vi "process waveplate positions.vi"(8 "error in (no error)":errorcluster, 11 "Channel in":refnum<class "SPARC4_Channel.lvclass">) -> (0 "error out":errorcluster, 3 "Channel out":refnum<class "SPARC4_Channel.lvclass">)   [LabVIEW 2018, in "SPARC4_Channel.lvclass"]
uses:
  SPARC4_Channel.lvclass
  SPARC4_Channel.lvclass/SPARC4_Channel.ctl
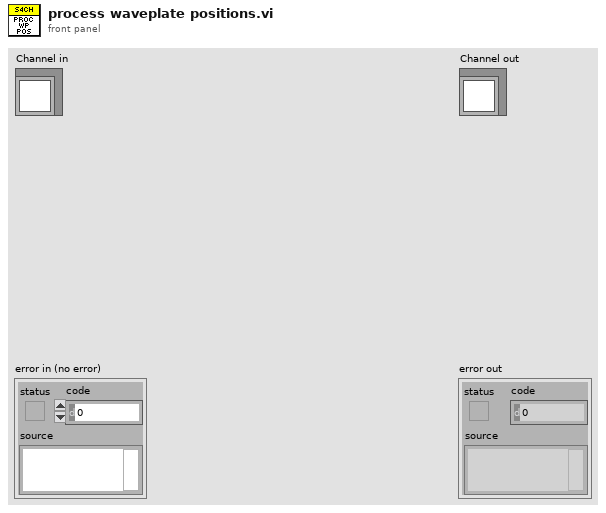
[diagram p1: front panel]
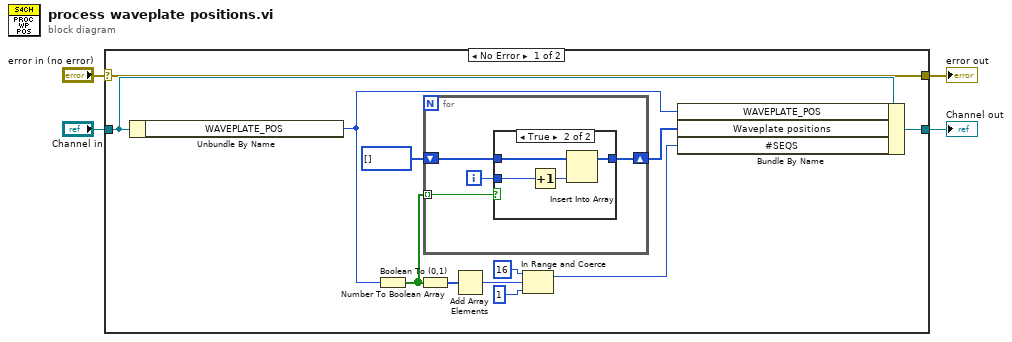
[diagram p0: block diagram]
diagram:
  n1 = case shown="No Error" "error in (no error)" {
    selector: "error in (no error)" -> [w5 w27]
    tunnel: [w5 w27] -> w1
    tunnel: [w15 w26] -> w2
    tunnel: "Channel in" -> [w16 w26]
    frame No Error {
      n2 = Unbundle By Name(w16) -> ("WAVEPLATE_POS"=w6:i32)
      n3 = Number To Boolean Array(number=w6) -> (Boolean array=w14:bool[])
      n4 = Boolean To (0,1)(Boolean=w14) -> (0, 1=w13:i16[])
      n5 = for {
        tunnel: w14 -> [w17] mode=indexing
        shift-right: [w18] -> w11
        shift-left: i32[] [] -> [w20]
        i -> [w19]
        n6 = case shown="True" w17 {
          tunnel: w20 -> [w21 w25]
          tunnel: w19 -> [_ w22]
          tunnel: [w21 w24] -> w18
          frame False {
          }
          frame True {
            n7 = Increment(x=w22) -> (x+1=w23:i32)
            n8 = Insert Into Array(array=w25, new element=w23) -> (w24:i32[])  [unwired: 1 in]
          }
        }
      }
      n9 = Add Array Elements(numeric array=w13) -> (sum=w10:i16)
      n10 = In Range and Coerce(upper limit=i16 16, x=w10, lower limit=i16 1) -> (coerced(x)=w7:i16)  [unwired: 1 out]
      n11 = Bundle By Name(cluster=w16, "WAVEPLATE_POS"=w6, "Waveplate positions"=w11, "#SEQS"=w7) -> (w15:refnum<class "SPARC4_Channel.lvclass">)
    }
    frame Error {
    }
  }
  "error out" <- w1
  "Channel out" <- w2
